vi "AxisLabel.vi"(1 "Axis":string(combo)="Gate") -> (0 "X Scale.Name Label.Text":string)   [LabVIEW 2011]
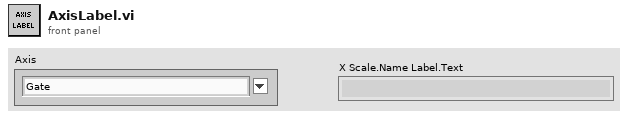
[diagram p1: front panel]
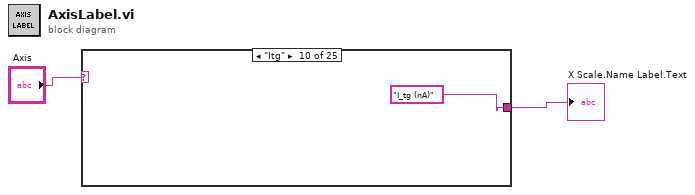
[diagram p0: block diagram]
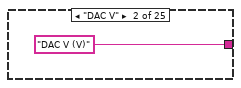
[diagram p3: hidden frame]
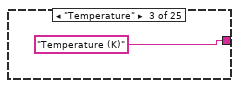
[diagram p4: hidden frame]
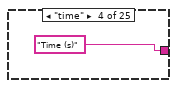
[diagram p5: hidden frame]
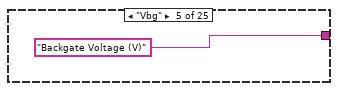
[diagram p6: hidden frame]
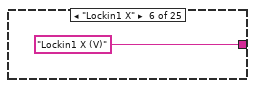
[diagram p7: hidden frame]
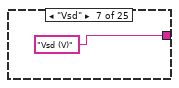
[diagram p8: hidden frame]
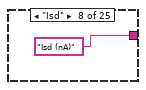
[diagram p9: hidden frame]
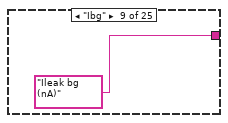
[diagram p10: hidden frame]
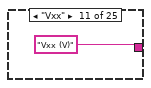
[diagram p11: hidden frame]
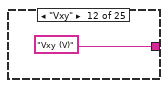
[diagram p12: hidden frame]
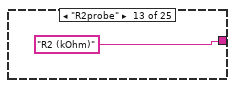
[diagram p13: hidden frame]
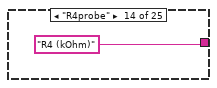
[diagram p14: hidden frame]
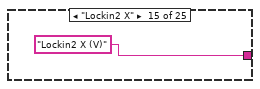
[diagram p15: hidden frame]
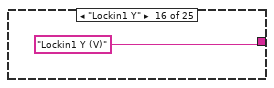
[diagram p16: hidden frame]
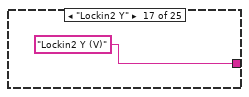
[diagram p17: hidden frame]
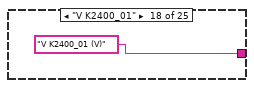
[diagram p18: hidden frame]
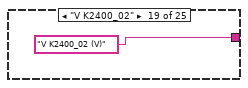
[diagram p19: hidden frame]
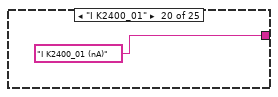
[diagram p20: hidden frame]
diagram:
  n1 = case shown="\"Itg\"" "Axis" {
    selector: "Axis" -> [w3 _ _ _ _ _ _ _ _ _ _ _ _ _ _ _ _ _ _ _ _ _ _ _ _]
    tunnel: [w3 "DAC V (V)" ("X Scale.Name Label.Text") "Temperature (K)" ("X Scale.Name Label.Text") "Time (s)" ("X Scale.Name Label.Text") "Backgate Voltage (V)" ("X Scale.Name Label.Text") "Lockin1 X (V)" ("X Scale.Name Label.Text") "Vsd (V)" ("X Scale.Name Label.Text") "Isd (nA)" ("X Scale.Name Label.Text") "Ileak bg (nA)" ("X Scale.Name Label.Text") "I_tg (nA)" ("X Scale.Name Label.Text") "Vxx (V)" ("X Scale.Name Label.Text") "Vxy (V)" ("X Scale.Name Label.Text") "R2 (kOhm)" ("X Scale.Name Label.Text") "R4 (kOhm)" ("X Scale.Name Label.Text") "Lockin2 X (V)" ("X Scale.Name Label.Text") "Lockin1 Y (V)" ("X Scale.Name Label.Text") "Lockin2 Y (V)" ("X Scale.Name Label.Text") "V K2400_01 (V)" ("X Scale.Name Label.Text") "V K2400_02 (V)" ("X Scale.Name Label.Text") "I K2400_01 (nA)" ("X Scale.Name Label.Text") "I K2400_02 (nA)" ("X Scale.Name Label.Text") "DMM1 (V)" ("X Scale.Name Label.Text") "Wavelength (nm)" ("X Scale.Name Label.Text") "DMM2 (V)" ("X Scale.Name Label.Text") "B (T)" ("X Scale.Name Label.Text")] -> w1
    frame "Formula1234", Default {
    }
    frame "DAC V" {
    }
    frame "Temperature" {
    }
    frame "time" {
    }
    frame "Vbg" {
    }
    frame "Lockin1 X" {
    }
    frame "Vsd" {
    }
    frame "Isd" {
    }
    frame "Ibg" {
    }
    frame "Itg" {
    }
    frame "Vxx" {
    }
    frame "Vxy" {
    }
    frame "R2probe" {
    }
    frame "R4probe" {
    }
    frame "Lockin2 X" {
    }
    frame "Lockin1 Y" {
    }
    frame "Lockin2 Y" {
    }
    frame "V K2400_01" {
    }
    frame "V K2400_02" {
    }
    frame "I K2400_01" {
    }
    frame "I K2400_02" {
    }
    frame "DMM1" {
    }
    frame "Wavelength" {
    }
    frame "DMM2" {
    }
    frame "B" {
    }
  }
  "X Scale.Name Label.Text" <- w1
